vi "Save_Trav_setup.vi"(0 "Work in Tunnel Coordinates?":T1, 1 "Trav Table":T2[](array[typedef]) {"Carrier_2 Q (l/min)" format="%#.2f"; "Row Duration (mins)" format="%#.1f"; "Row No" min=0; "Trace Gas Concentration (%)" min=0.0 format="%#_4f"; "Carrier_1 Q (l/min)" format="%#.2f"; "Tunnel Speed" format="%#.2f"; "Start X" format="%#.2f"; "Start Y" format="%#.2f"; "Start Z" format="%#.2f"; "End X" format="%#.2f"; "End Y" format="%#.2f"; "End Z" format="%#.2f"; "Averaging time (min)" min=0.0 format="%#.2f"}, 2 "Fast Plotting?":bool, 3 "Jump Bad Positions":bool, 4 "Setup filename":path) -> (5 "Trav Table Out":T2[](array[typedef]) {"Carrier_2 Q (l/min)" format="%#.2f"; "Row Duration (mins)" format="%#.1f"; "Row No" min=0; "Trace Gas Concentration (%)" min=0.0 format="%#_4f"; "Carrier_1 Q (l/min)" format="%#.2f"; "Tunnel Speed" format="%#.2f"; "Start X" format="%#.2f"; "Start Y" format="%#.2f"; "Start Z" format="%#.2f"; "End X" format="%#.2f"; "End Y" format="%#.2f"; "End Z" format="%#.2f"; "Averaging time (min)" min=0.0 format="%#.2f"})   [LabVIEW 2016]
uses:
  Traverse_cluster.ctl
  Spacing.ctl
  Controls/Multi_run_mode.ctl
  Controls/Tunnel_Coordinates.ctl
  File/Setup_Filetype.ctl
panel:
  # "X           Y            Z"
  # "Start"
  # "End"
  # "X           Y            Z"
  # "Start"
  # "End"
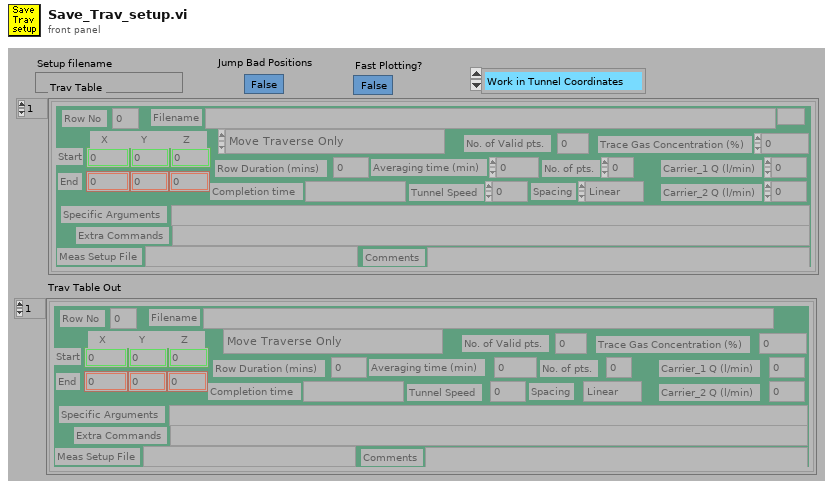
[diagram p1: front panel]
types:
  T1 = typedef "Tunnel_Coordinates.ctl" = enum16{"Work in Tunnel Coordinates", "Work in Model Coordinates"}
  T2 = typedef "Traverse_cluster.ctl" = cluster{"Start X":sgl, "Start Y":sgl, "Start Z":sgl, "End X":sgl, "End Y":sgl, "End Z":sgl, "No. of pts.":i32, "Spacing":T3, "Filename":path, "Tunnel Speed":dbl, "Averaging time (min)":dbl, "Extra Commands":string, "Carrier_1 Q (l/min)":dbl, "Carrier_2 Q (l/min)":dbl, "Trace Gas Concentration (%)":dbl, "Specific Arguments":string, "Comments":string, "Row No":i32, "Row Type Selector":T4, "Completion time":string, "Row Duration (mins)":dbl, "No. of Valid pts.":i32, "Meas Setup File":string}
  T3 = typedef "Spacing.ctl" = enum16{"Linear", "Log", "Gauss", "Specified", "N/A"}
  T4 = typedef "Multi_run_mode.ctl" = enum16{"Move Traverse Only", "Set Tunnel Speed Only", "Set Source Only", "Set Measurement Conditions", "Single Measurement", "Vertical Profile", "Lateral Profile", "Longitudinal Profile", "Explore Volume", "Multi-Axis Profile", "Auto Calibrate", "Meas Fast FID Bkgnd", "Check Beam Power", "Scanning Valve Measurement", "Run VI Named:", "Set ADAM Ch", "Wait (minutes)", "Send Message", "Synchronize With:", "Fall Back to this Row", "Turn Off Row Repeating", "Blank Row", "Traverse 3D Volume"}
  T5 = enum16{"All Channel Names", "Valid Channel Names"}
  T6 = typedef "Setup_Filetype.ctl" = enum16{"Measurement Setups", "Calibration Setups", "General", "Results File Plotter Setups", "Speed Calib Tweaks"}
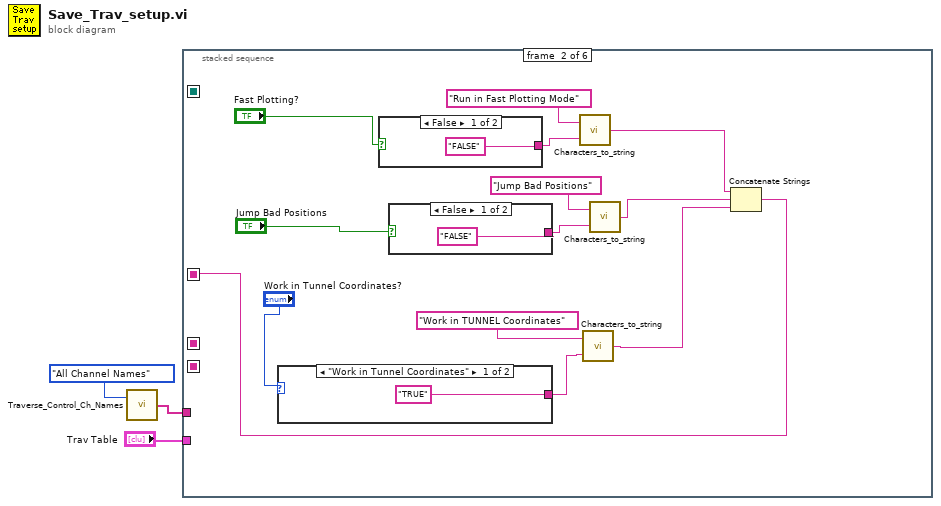
[diagram p0: block diagram]
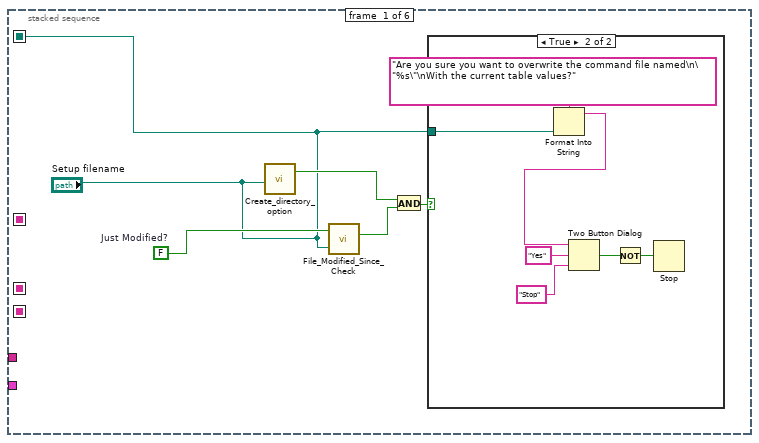
[diagram p2: hidden frame]
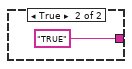
[diagram p4: hidden frame]
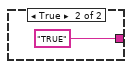
[diagram p5: hidden frame]
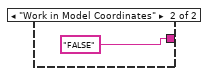
[diagram p6: hidden frame]
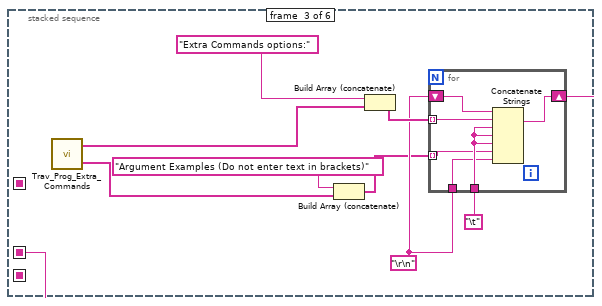
[diagram p7: hidden frame]
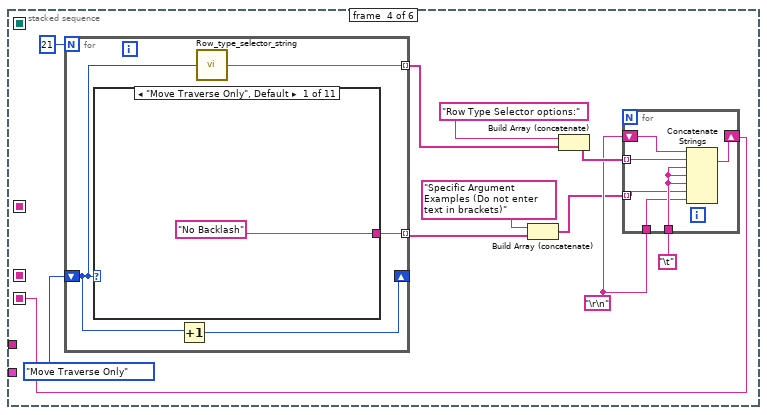
[diagram p8: hidden frame]
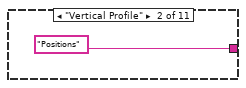
[diagram p9: hidden frame]
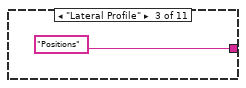
[diagram p10: hidden frame]
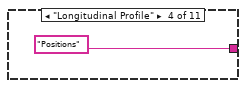
[diagram p11: hidden frame]
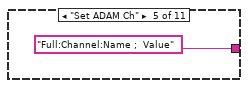
[diagram p12: hidden frame]
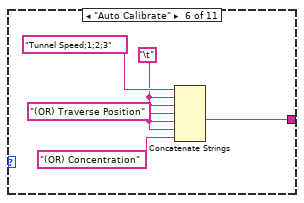
[diagram p13: hidden frame]
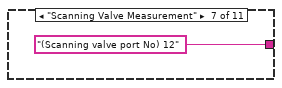
[diagram p14: hidden frame]
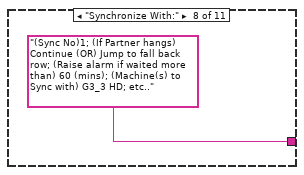
[diagram p15: hidden frame]
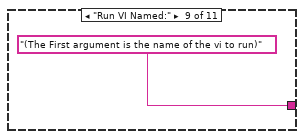
[diagram p16: hidden frame]
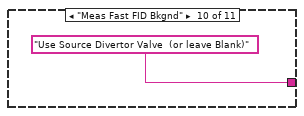
[diagram p17: hidden frame]
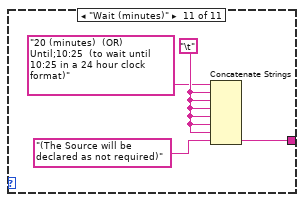
[diagram p18: hidden frame]
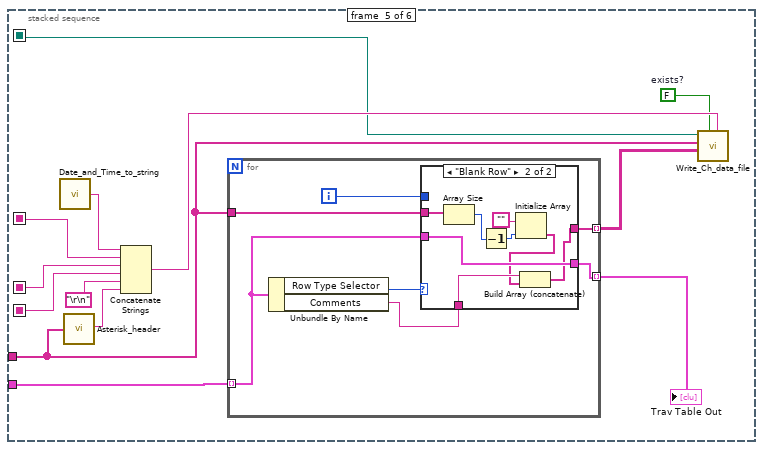
[diagram p19: hidden frame]
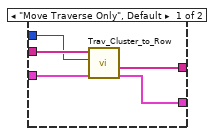
[diagram p20: hidden frame]
diagram:
  n1 = call "Traverse_Control_Ch_Names.vi"("Mode"=T5."All Channel Names") -> ("Channel names"=w3:string[])  [unwired: 1 in]
  n2 = stacked-sequence {
    seq-local: [_ w28 _ _ _ _] -> [_ _ _ _ w97 _]
    seq-local: [_ _ w41 _ _ _] -> [_ _ _ _ w99 _]
    seq-local: [_ _ _ w54 _ _] -> [_ _ _ _ w96 _]
    seq-local: ["Setup filename" _ _ _ _ _] -> [_ _ _ _ w90 w128]
    tunnel: w3 -> [_ _ _ _ w95 _]
    tunnel: "Trav Table" -> [_ _ _ _ w89 _]
    frame #0 {
      w5 = FALSE  # Just Modified?
      n3 = call "Create_directory_option.vi"("Filename"="Setup filename") -> ("Path is to existing File"=w7:bool)  [unwired: 1 out]
      n4 = call "File_Modified_Since_Check.vi"("Pathname"="Setup filename", "Just Modified?"=w5) -> ("Modified?"=w8:bool)
      n5 = And(x=w7, y=w8) -> (x .and. y?=w6:bool)
      n6 = case shown="True" w6 {
        tunnel: "Setup filename" -> [_ w15]
        frame False {
        }
        frame True {
          n7 = Format Into String(format string="Are you sure you want to overwrite the command file named\n\"%s\"\nWith the current table values?" ("Format String"), w15) -> (resulting string=w13:string)  [unwired: 2 in, 1 out]
          n8 = Two Button Dialog(message=w13, 1:"Stop" ("F button name (\"Cancel\")"), 2:"Yes" ("T button name (\"OK\")")) -> (T button?=w10:bool)
          n9 = Not(x=w10) -> (.not. x?=w9:bool)
          n10 = Stop(stop? (T)=w9) -> ()
        }
      }
    }
    frame #1 {
      n11 = case shown="\"Work in Tunnel Coordinates\"" "Work in Tunnel Coordinates?" {
        tunnel: ["TRUE" "FALSE" ("f")] -> w24
        frame "Work in Tunnel Coordinates" {
        }
        frame "Work in Model Coordinates" {
        }
      }
      n12 = case shown="False" "Fast Plotting?" {
        tunnel: ["FALSE" ("f") "TRUE"] -> w18
        frame False {
        }
        frame True {
        }
      }
      n13 = case shown="False" "Jump Bad Positions" {
        tunnel: ["FALSE" ("f") "TRUE"] -> w22
        frame False {
        }
        frame True {
        }
      }
      n14 = call "Characters_to_string.vi"("Characters to write"=w18, "Label for characters"="Run in Fast Plotting Mode") -> ("Output string"=w16:string)
      n15 = call "Characters_to_string.vi"("Characters to write"=w24, "Label for characters"="Work in TUNNEL Coordinates") -> ("Output string"=w26:string)
      n16 = call "Characters_to_string.vi"("Characters to write"=w22, "Label for characters"="Jump Bad Positions") -> ("Output string"=w20:string)
      n17 = Concatenate Strings(w16, w20, w26) -> (w28:string)
    }
    frame #2 {
      w42 = "\r\n"
      n18 = call "Trav_Prog_Extra_Commands.vi"() -> ("Extra Commands Array"=w39:string[], "Argument Examples"=w38:string[])  [unwired: 1 out]
      n19 = Build Array (concatenate)("Argument Examples (Do not enter text in brackets)" ("Substring"), w38) -> (w37:string[])
      n20 = Build Array (concatenate)("Extra Commands options:", w39) -> (w43:string[])
      n21 = for {
        shift-right: [w47] -> w41
        shift-left: w42 -> [w48]
        tunnel: w43 -> [w49] mode=indexing
        tunnel: w42 -> [w44]
        tunnel: w37 -> [w45] mode=indexing
        tunnel: "\t" -> [w46]
        n22 = Concatenate Strings(w48, w49, w46, w46, w46, w45, w44) -> (w47:string)
      }
    }
    frame #3 {
      w59 = "\r\n"
      n23 = for {
        N: 21 -> [_]
        shift-right: [w64] -> _
        shift-left: Multi_run_mode."Move Traverse Only" ("Mode") -> [w63]
        tunnel: [w62] -> w52 mode=indexing
        tunnel: [w61] -> w51 mode=indexing
        n24 = case shown="\"Move Traverse Only\", Default" w63 {
          tunnel: ["No Backlash" "Positions" "Positions" "Positions" "Full:Channel:Name ;  Value" w74 "(Scanning valve port No) 12" "(Sync No)1; (If Partner hangs) Continue (OR) Jump to fall back row; (Raise alarm if waited more than) 60 (mins); (Machine(s) to Sync with) G3_3 HD; etc.." "(The First argument is the name of the vi to run)" "Use Source Divertor Valve  (or leave Blank)" w82] -> w61
          frame "Move Traverse Only", Default {
          }
          frame "Vertical Profile" {
          }
          frame "Lateral Profile" {
          }
          frame "Longitudinal Profile" {
          }
          frame "Set ADAM Ch" {
          }
          frame "Auto Calibrate" {
            w71 = "\t"
            n25 = Concatenate Strings("Tunnel Speed;1;2;3", w71, w71, "(OR) Traverse Position", w71, w71, "(OR) Concentration") -> (w74:string)
          }
          frame "Scanning Valve Measurement" {
          }
          frame "Synchronize With:" {
          }
          frame "Run VI Named:" {
          }
          frame "Meas Fast FID Bkgnd" {
          }
          frame "Wait (minutes)" {
            w80 = "\t"
            n26 = Concatenate Strings("20 (minutes)  (OR) Until;10:25  (to wait until 10:25 in a 24 hour clock format)" ("Substring"), w80, w80, w80, w80, w80, w80, "(The Source will be declared as not required)") -> (w82:string)
          }
        }
        n27 = Increment(x=w63) -> (x+1=w64:T4)
        n28 = call "Row_type_selector_string.vi"("Mode"=w63) -> ("Output string"=w62:string)
      }
      n29 = Build Array (concatenate)("Specific Argument Examples (Do not enter text in brackets)" ("Substring"), w51) -> (w57:string[])
      n30 = Build Array (concatenate)("Row Type Selector options:", w52) -> (w60:string[])
      n31 = for {
        shift-right: [w86] -> w54
        shift-left: w59 -> [w87]
        tunnel: w60 -> [w88] mode=indexing
        tunnel: w59 -> [w83]
        tunnel: w57 -> [w84] mode=indexing
        tunnel: "\t" -> [w85]
        n32 = Concatenate Strings(w87, w88, w85, w85, w85, w84, w83) -> (w86:string)
      }
    }
    frame #4 {
      w100 = FALSE  # exists?
      n33 = call "Date_and_Time_to_string.vi"() -> ("Date and time (spreadsheet)"=w98:string)
      n34 = call "Asterisk_header.vi"("Channel names"=w95) -> ("Header string"=w91:string)
      n35 = Concatenate Strings(w98, w97, w99, w96, "\r\n", w91) -> (w101:string)
      n36 = for {
        tunnel: w95 -> [w108]
        tunnel: w89 -> [w104] mode=indexing
        tunnel: [w107] -> w94 mode=indexing
        tunnel: [w106] -> w93 mode=indexing
        i -> [w105]
        n37 = Unbundle By Name(w104) -> ("Row Type Selector"=w103:T4, "Comments"=w102:string)
        n38 = case shown="\"Blank Row\"" w103 {
          tunnel: w108 -> [w113 w120]
          tunnel: [w112 w114] -> w107
          tunnel: [w111 w121] -> w106
          tunnel: w105 -> [w110 _]
          tunnel: w104 -> [w109 w121]
          tunnel: w102 -> [_ w116]
          frame "Move Traverse Only", Default {
            n39 = call "Trav_Cluster_to_Row.vi"("Traverse line in"=w109, "Row Number"=w110, "Channel names"=w113) -> ("Traverse line Out"=w111:T2, "Channel Values Out"=w112:string[])  [unwired: 3 out]
          }
          frame "Blank Row" {
            n40 = Array Size(array=w120) -> (size(s)=w118:i32)
            n41 = Decrement(x=w118) -> (x-1=w117:i32)
            n42 = Initialize Array("", w117) -> (w115:string[])
            n43 = Build Array (concatenate)(w116, w115) -> (w114:string[])
          }
        }
      }
      "Trav Table Out" <- w93
      n44 = call "Write_Ch_data_file.vi"("Header string"=w101, "exists?"=w100, "Channel Values"=w94, "Channel names"=w95, "Filename"=w90) -> ()  [unwired: 3 in, 4 out]
    }
    frame #5 {
      w125 = FALSE  # append to file? (new file:F)
      w126 = FALSE  # advisory dialog? (display:T)
      w129 = TRUE  # Just Modified?
      n45 = call "Setup_Filepath.vi"("Setup File Type"=Setup_Filetype."General", "Filename in"="Multi_Run_Filename.txt" ("name or relative path")) -> ("Filename Out"=w122:path)  [unwired: 1 out]
      n46 = Path To String(path=w128) -> (string=w127:string)
      n47 = call "Write_Characters_To_File.vi"("file path (dialog if empty)"=w122, "advisory dialog? (display:T)"=w126, "character string"=w127, "append to file? (new file:F)"=w125) -> ()  [unwired: 1 in, 4 out]
      n48 = call "File_Modified_Since_Check.vi"("Pathname"=w128, "Just Modified?"=w129) -> ()  [unwired: 1 out]
    }
  }
